vi "Post-Arm.vi"(8 "error in (no error)":errorcluster, 11 "Pulse Driver in":refnum<class "Pulse Driver.lvclass">) -> (0 "error out":errorcluster, 2 "Armed configuration":refnum<class "Start Stream Result.lvclass">, 3 "Pulse Driver out":refnum<class "Pulse Driver.lvclass">)   [LabVIEW 2024, in "Pulse Driver.lvclass"]
uses:
  Pulse Driver.lvclass
  C:/GitHub/NHMFL_Core/Libraries/Instruments/Instrument Driver/Instrument Driver.lvclass
  Results/Start Stream Result/Start Stream Result.lvclass
  C:/GitHub/NHMFL_Core/Libraries/Instruments/Results/Acquired Result/Acquired Result.lvclass
  Pulse Driver.lvclass/Pulse Driver.ctl
  Instrument Driver/Instrument Driver.lvclass/Instrument Driver.ctl
  Results/Acquired Result/Acquired Result.lvclass/Acquired Result.ctl
  Results/Start Stream Result/Start Stream Result.lvclass/Start Stream Result.ctl
  Write t0.vi
  Write dt.vi
  Read Set timing from UI.vi
  Read t0.vi
  Read dt.vi
  Instrument Driver/Read Recorder name.vi
  Results/Acquired Result/Write Channels.vi
  Results/Start Stream Result/Write t0.vi
  Results/Start Stream Result/Write dt.vi
  Results/Start Stream Result/Write Scaling coefficients.vi
  Results/Acquired Result/Write Sender.vi
  Results/Acquired Result/Write Group.vi
  Write Current read position.vi
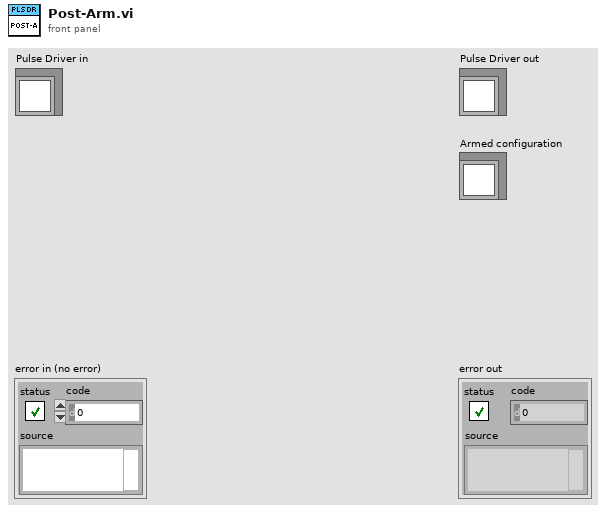
[diagram p1: front panel]
types:
  T1 = typedef "Pusle Driver Configuration.ctl" = cluster{"Post-trigger delay":dbl, "Post-trigger duration":dbl, "Rate":dbl, "Ranges":dbl[], "Re-name channels":string[], "Active channels":string, "External clock":bool}
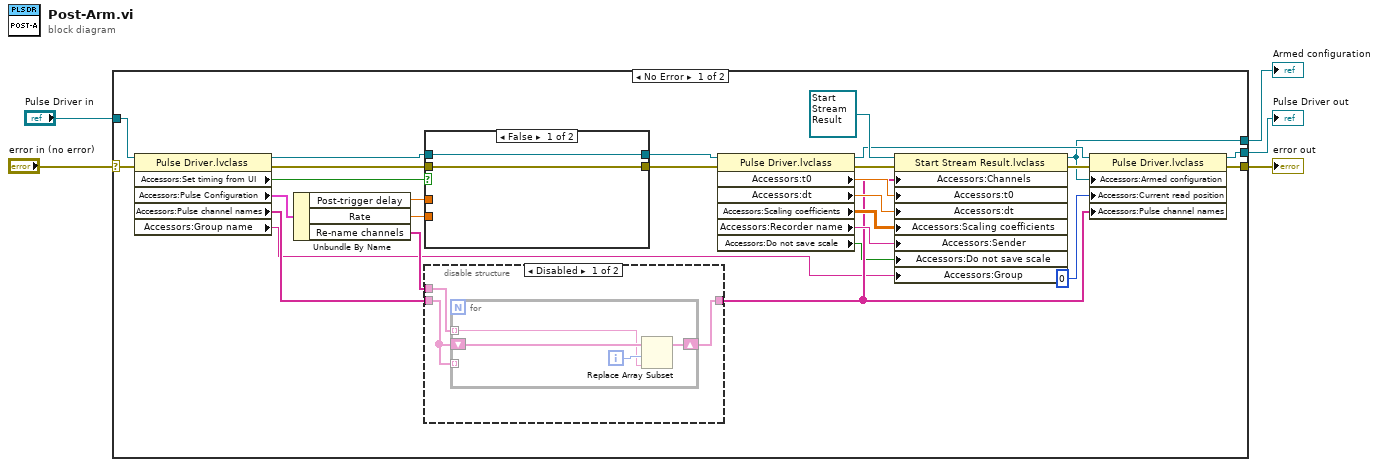
[diagram p0: block diagram]
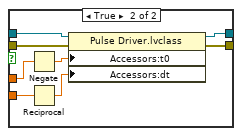
[diagram p3: hidden frame]
diagram:
  n1 = case shown="No Error" "error in (no error)" {
    selector: "error in (no error)" -> [w23 w52]
    tunnel: [w12 w52] -> w4
    tunnel: [w13 w51] -> w2
    tunnel: "Pulse Driver in" -> [w24 w51]
    tunnel: [w8 _] -> w1
    frame No Error {
      n2 = property class="Pulse Driver.lvclass"(reference=w24, error in=w23) -> (reference out=w30:refnum<class "Pulse Driver.lvclass">, error out=w29:errorcluster, "Accessors:Set timing from UI"=w25:bool, "Accessors:Pulse Configuration"=w26:T1, "Accessors:Pulse channel names"=w27:string[], "Accessors:Group name"=w6:string)
      n3 = Unbundle By Name(w26) -> ("Post-trigger delay"=w32:dbl, "Rate"=w31:dbl, "Re-name channels"=w28:string[])
      n4 = case shown="False" w25 {
        tunnel: w32 -> [_ w50]
        tunnel: w31 -> [_ w49]
        tunnel: w30 -> [w42 w46]
        tunnel: [w42 w45] -> w11
        tunnel: [w41 w44] -> w10
        tunnel: w29 -> [w41 w43]
        frame False {
        }
        frame True {
          n5 = Negate(x=w50) -> (-x=w48:dbl)
          n6 = Reciprocal(x=w49) -> (1/x=w47:dbl)
          n7 = property class="Pulse Driver.lvclass"(reference=w46, error in=w43, "Accessors:t0"=w48, "Accessors:dt"=w47) -> (reference out=w45:refnum<class "Pulse Driver.lvclass">, error out=w44:errorcluster)
        }
      }
      n8 = disable-structure shown="Disabled" {
        disable-tunnel: [w35 w40] -> w16
        disable-tunnel: w28 -> [w34 _]
        disable-tunnel: w27 -> [w33 w40]
        frame Disabled {
          n9 = for {
            tunnel: w34 -> [w37] mode=indexing
            shift-right: [w36] -> w35
            shift-left: w33 -> [w39]
            tunnel: w33 -> [_] mode=indexing
            i -> [w38]
            n10 = Replace Array Subset(array=w39, new element=w37, index=w38) -> (w36:string[])
          }
        }
        frame Enabled {
        }
      }
      n11 = property class="Pulse Driver.lvclass"(reference=w11, error in=w10) -> (reference out=w14:refnum<class "Pulse Driver.lvclass">, error out=w21:errorcluster, "Accessors:t0"=w18:dbl, "Accessors:dt"=w19:dbl, "Accessors:Scaling coefficients"=w20:dbl[][], "Accessors:Recorder name"=w22:string, "Accessors:Do not save scale"=w7:bool)
      n12 = property class="Start Stream Result.lvclass"(reference=refnum<class "Start Stream Result.lvclass"> refnum ("Start Stream Result.lvclass"), error in=w21, "Accessors:Channels"=w16, "Accessors:t0"=w18, "Accessors:dt"=w19, "Accessors:Scaling coefficients"=w20, "Accessors:Sender"=w22, "Accessors:Do not save scale"=w7, "Accessors:Group"=w6) -> (reference out=w8:refnum<class "Start Stream Result.lvclass">, error out=w15:errorcluster)
      n13 = property class="Pulse Driver.lvclass"(reference=w14, error in=w15, "Accessors:Armed configuration"=w8, "Accessors:Current read position"=0 ("Current read position"), "Accessors:Pulse channel names"=w16) -> (reference out=w13:refnum<class "Pulse Driver.lvclass">, error out=w12:errorcluster)
    }
    frame Error {
    }
  }
  "error out" <- w4
  "Pulse Driver out" <- w2
  "Armed configuration" <- w1
